vi "Update Register Values - 321.vi"(8 "error in (no error)":errorcluster, 11 "Register Value":variant) -> (0 "error out":errorcluster, 3 "Updated Register Values":T1[](array[typedef]) {"Data Type" format="%.0x"})   [LabVIEW 2019, in "FPGA Addon Shared.lvlib"]
uses:
  FPGA Addon Shared.lvlib
  Types/Register Information.ctl
  Types/FPGA Addon Data Type.ctl
  APIs/FPGA Register IO/TypeDefs/FXP Configuration.ctl
  <vilib>/fxp/LVFixedPointRepBitsTypeDef.ctl
  <vilib>/fxp/LVFixedPointRepRangeTypeDef.ctl
  <vilib>/Utility/Data Type/NI_Data Type.lvlib
  APIs/FPGA Register IO/FPGA Register IO.lvlib
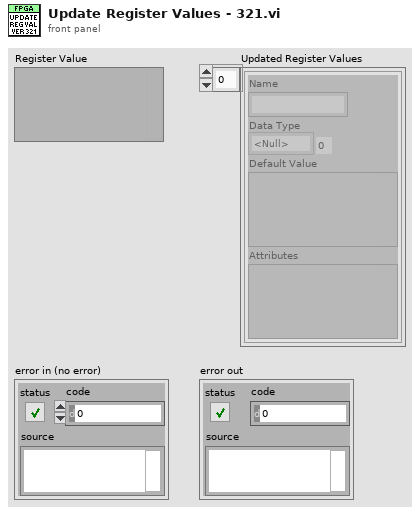
[diagram p1: front panel]
types:
  T1 = typedef "FPGA Addon Shared.lvlib/Register Information.ctl" = cluster{"Name":string, "Data Type":T2, "Default Value":variant, "Attributes":variant}
  T2 = typedef "FPGA Addon Shared.lvlib/FPGA Addon Data Type.ctl" = enum8{"<Null>", "I8", "I16", "I32", "I64", "U8", "U16", "U32", "U64", "SGL", "Boolean", "Analog PWM In Settings", "Analog PWM In", "Digital PWM In Settings", "Digital PWM In", "Digital PWM Out", "Sine Out", "FXP", "FXP+/-24.5", "FXP+/-16.5", "FXP+/-32.8", "FXP+/-64.32", "FXP+/-16.7", "FXP+/-20.5", "FXP+/-27.5", "FXP+/-32.16", "FXP+16.3", "FXP+18.3", "Digital Static In", "Digital Static Out", "Digital Static In Settings", "Digital WSS Out", "Quad Encoder Settings", "Quad Encoder In", "Group"}
  T3 = cluster{"Name":string, "Data Type":enum8{"<Null>", "I8", "I16", "I32", "I64", "U8", "U16", "U32", "U64", "SGL", "Boolean", "Analog PWM In Settings", "Analog PWM In", "Digital PWM In Settings", "Digital PWM In", "Digital PWM Out", "Sine Out", "FXP+/-24.5", "FXP+/-16.5", "FXP+/-32.8", "FXP+/-64.32", "FXP+/-16.7", "FXP+/-20.5", "FXP+/-27.5", "FXP+/-32.16", "FXP+16.3", "FXP+18.3", "Digital Static In", "Digital Static Out", "Digital Static In Settings", "Digital WSS Out", "Quad Encoder Settings", "Quad Encoder In", "Group"}, "Default Value":variant}[]
  T4 = typedef "FPGA Register IO.lvlib/FXP Configuration.ctl" = cluster{"FXP Representation":T5, "FXP Range":T6}
  T5 = typedef "LVFixedPointRepBitsTypeDef.ctl" = cluster{"Signed":bool, "Word Length":u32, "Integer Word Length":i32}
  T6 = typedef "LVFixedPointRepRangeTypeDef.ctl" = cluster{"Range Min":dbl, "Range Max":dbl, "Delta":dbl}
  T7 = enum8{"<Null>", "I8", "I16", "I32", "I64", "U8", "U16", "U32", "U64", "SGL", "Boolean", "Analog PWM In Settings", "Analog PWM In", "Digital PWM In Settings", "Digital PWM In", "Digital PWM Out", "Sine Out", "FXP+/-24.5", "FXP+/-16.5", "FXP+/-32.8", "FXP+/-64.32", "FXP+/-16.7", "FXP+/-20.5", "FXP+/-27.5", "FXP+/-32.16", "FXP+16.3", "FXP+18.3", "Digital Static In", "Digital Static Out", "Digital Static In Settings", "Digital WSS Out", "Quad Encoder Settings", "Quad Encoder In", "Group"}
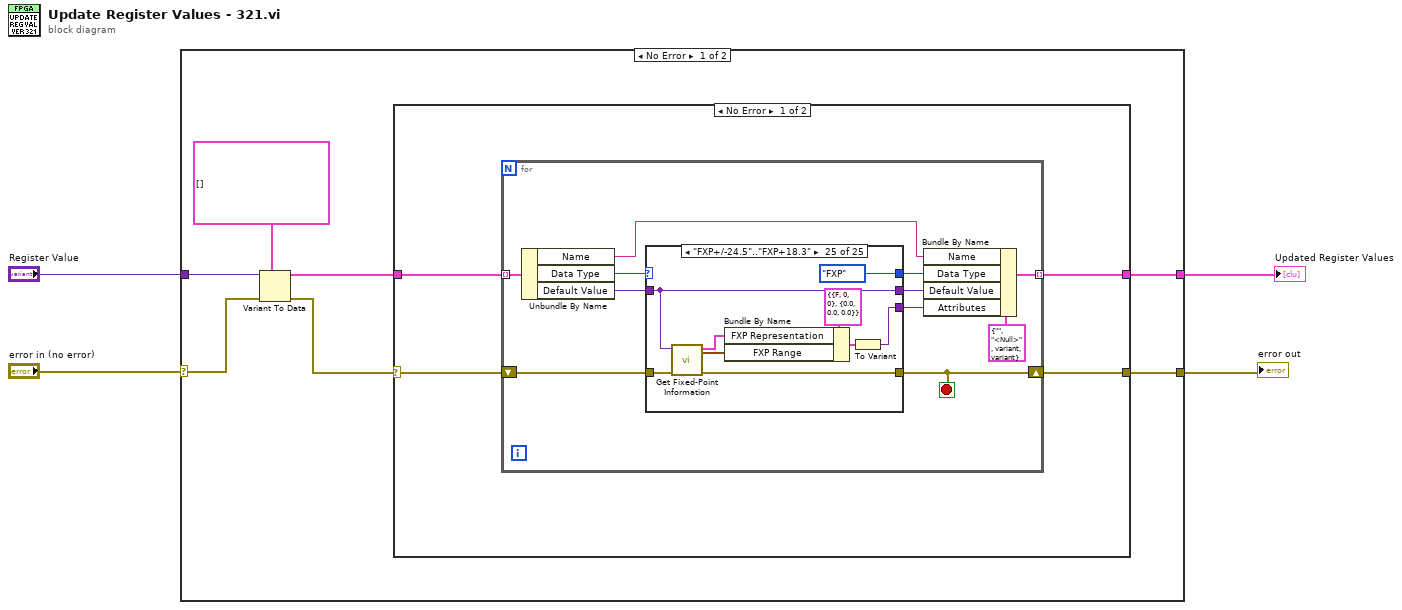
[diagram p0: block diagram]
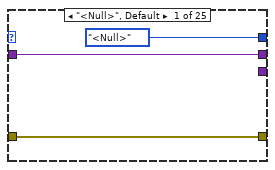
[diagram p2: hidden frame]
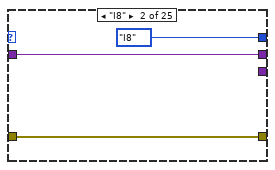
[diagram p3: hidden frame]
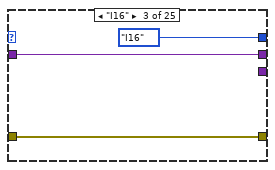
[diagram p4: hidden frame]
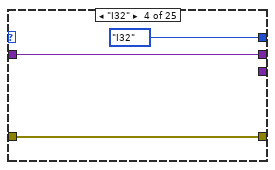
[diagram p5: hidden frame]
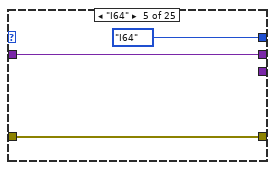
[diagram p6: hidden frame]
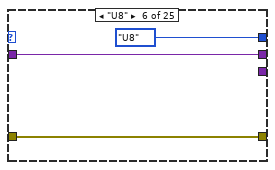
[diagram p7: hidden frame]
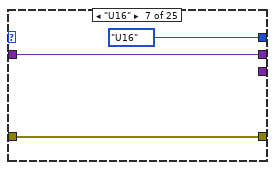
[diagram p8: hidden frame]
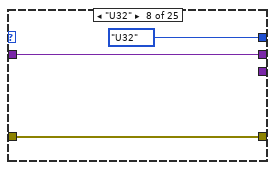
[diagram p9: hidden frame]
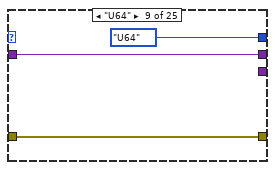
[diagram p10: hidden frame]
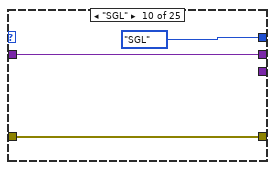
[diagram p11: hidden frame]
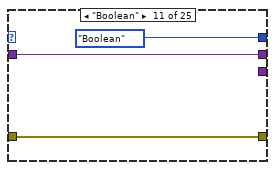
[diagram p12: hidden frame]
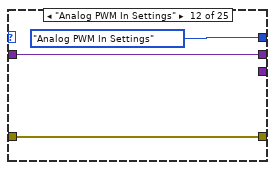
[diagram p13: hidden frame]
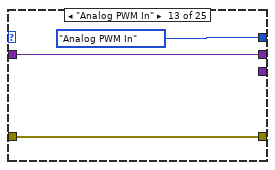
[diagram p14: hidden frame]
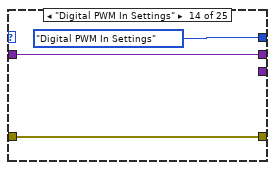
[diagram p15: hidden frame]
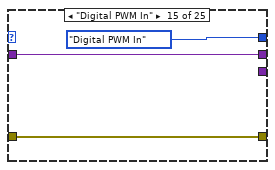
[diagram p16: hidden frame]
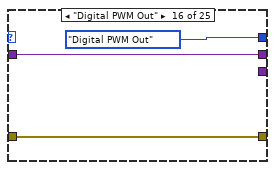
[diagram p17: hidden frame]
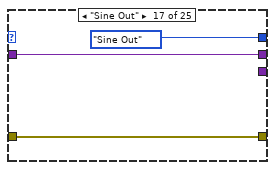
[diagram p18: hidden frame]
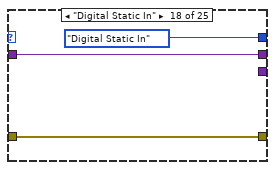
[diagram p19: hidden frame]
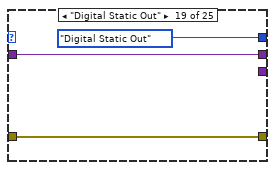
[diagram p20: hidden frame]
diagram:
  n1 = case shown="No Error" "error in (no error)" {
    selector: "error in (no error)" -> [w7 w112]
    tunnel: [w10 _] -> w4
    tunnel: "Register Value" -> [w8 _]
    tunnel: [w5 w112] -> w1
    frame No Error {
      n2 = Variant To Data(error in=w7, type=T3 [] ("Available Registers 2"), Variant=w8) -> (data=w9:T3, error out=w6:errorcluster)
      n3 = case shown="No Error" w6 {
        selector: w6 -> [w13 w111]
        tunnel: [w15 _] -> w10
        tunnel: w9 -> [w14 _]
        tunnel: [w12 w111] -> w5
        frame No Error {
          n4 = for {
            tunnel: w14 -> [w26] mode=indexing
            tunnel: [w24] -> w15 mode=indexing
            shift-right: [w18] -> w12
            shift-left: w13 -> [w19]
            stop <- w18 stop-if-true
            n5 = Unbundle By Name(w26) -> ("Name"=w17:string, "Data Type"=w23:T7, "Default Value"=w22:variant)
            n6 = case shown="\"FXP+/-24.5\"..\"FXP+18.3\"" w23 {
              tunnel: [FPGA_Addon_Data_Type."<Null>" ("Data Type") FPGA_Addon_Data_Type."I8" ("Data Type") FPGA_Addon_Data_Type."I16" ("Data Type") FPGA_Addon_Data_Type."I32" ("Data Type") FPGA_Addon_Data_Type."I64" ("Data Type") FPGA_Addon_Data_Type."U8" ("Data Type") FPGA_Addon_Data_Type."U16" ("Data Type") FPGA_Addon_Data_Type."U32" ("Data Type") FPGA_Addon_Data_Type."U64" ("Data Type") FPGA_Addon_Data_Type."SGL" ("Data Type") FPGA_Addon_Data_Type."Boolean" ("Data Type") FPGA_Addon_Data_Type."Analog PWM In Settings" ("Data Type") FPGA_Addon_Data_Type."Analog PWM In" ("Data Type") FPGA_Addon_Data_Type."Digital PWM In Settings" ("Data Type") FPGA_Addon_Data_Type."Digital PWM In" ("Data Type") FPGA_Addon_Data_Type."Digital PWM Out" ("Data Type") FPGA_Addon_Data_Type."Sine Out" ("Data Type") FPGA_Addon_Data_Type."Digital Static In" ("Data Type") FPGA_Addon_Data_Type."Digital Static Out" ("Data Type") FPGA_Addon_Data_Type."Digital Static In Settings" ("Data Type") FPGA_Addon_Data_Type."Digital WSS Out" ("Data Type") FPGA_Addon_Data_Type."Quad Encoder Settings" ("Data Type") FPGA_Addon_Data_Type."Quad Encoder In" ("Data Type") FPGA_Addon_Data_Type."Group" ("Data Type") FPGA_Addon_Data_Type."FXP" ("Data Type")] -> w20
              tunnel: [w28 w31 w34 w37 w40 w43 w46 w49 w52 w55 w58 w61 w64 w67 w70 w73 w76 w79 w82 w85 w88 w91 w94 w99 w104] -> w21
              tunnel: w22 -> [w28 w31 w34 w37 w40 w43 w46 w49 w52 w55 w58 w61 w64 w67 w70 w73 w76 w79 w82 w85 w88 w91 w94 w98 w104]
              tunnel: w19 -> [w27 w30 w33 w36 w39 w42 w45 w48 w51 w54 w57 w60 w63 w66 w69 w72 w75 w78 w81 w84 w87 w90 w93 w97 w103]
              tunnel: [w27 w30 w33 w36 w39 w42 w45 w48 w51 w54 w57 w60 w63 w66 w69 w72 w75 w78 w81 w84 w87 w90 w93 w96 w102] -> w18
              tunnel: [_ _ _ _ _ _ _ _ _ _ _ _ _ _ _ _ _ _ _ _ _ _ _ _ w105] -> w16
              frame "<Null>", Default {
              }
              frame "I8" {
              }
              frame "I16" {
              }
              frame "I32" {
              }
              frame "I64" {
              }
              frame "U8" {
              }
              frame "U16" {
              }
              frame "U32" {
              }
              frame "U64" {
              }
              frame "SGL" {
              }
              frame "Boolean" {
              }
              frame "Analog PWM In Settings" {
              }
              frame "Analog PWM In" {
              }
              frame "Digital PWM In Settings" {
              }
              frame "Digital PWM In" {
              }
              frame "Digital PWM Out" {
              }
              frame "Sine Out" {
              }
              frame "Digital Static In" {
              }
              frame "Digital Static Out" {
              }
              frame "Digital Static In Settings" {
              }
              frame "Digital WSS Out" {
              }
              frame "Quad Encoder Settings" {
              }
              frame "Quad Encoder In" {
              }
              frame "Group" {
                n7 = call "Update Register Values - 321.vi"("error in (no error)"=w97, "Register Value"=w98) -> ("error out"=w96:errorcluster, "Updated Register Values"=w100:T1[])  [unwired: 8 in]
                n8 = To Variant(anything=w100) -> (Variant=w99:variant)
              }
              frame "FXP+/-24.5".."FXP+18.3" {
                n9 = call <vilib>:"Get Fixed-Point Information.vi"("error in (no error)"=w103, "variant"=w104) -> ("error out"=w102:errorcluster, "FXP range"=w108:T6, "FXP representation"=w107:T5)  [unwired: 6 in, 1 out]
                n10 = Bundle By Name(cluster=T4 {"FXP Representation"={"Signed"=FALSE, "Word Length"=0, "Integer Word Length"=0}, "FXP Range"={"Range Min"=0.0, "Range Max"=0.0, "Delta"=0.0}} ("FXP Configuration"), "FXP Representation"=w107, "FXP Range"=w108) -> (w109:T4)
                n11 = To Variant(anything=w109) -> (Variant=w105:variant)
              }
            }
            n12 = Bundle By Name(cluster=T1 {"Name"="", "Data Type"=enum."<Null>", "Default Value"=variant(refnum<class> refnum), "Attributes"=variant}, "Name"=w17, "Data Type"=w20, "Default Value"=w21, "Attributes"=w16) -> (w24:T1)
          }
        }
        frame Error {
        }
      }
    }
    frame Error {
    }
  }
  "Updated Register Values" <- w4
  "error out" <- w1
